vi "Unsubscribe from Topic.vi"(8 "error in (no error)":errorcluster, 9 "Topic":string, 10 "Subscriber Enq":refnum<class "Message Enqueuer.lvclass">, 11 "Publisher Actor in":refnum<class "Publisher Actor.lvclass">) -> (0 "error out":errorcluster, 3 "Publisher Actor out":refnum<class "Publisher Actor.lvclass">)   [LabVIEW 2021, in "Publisher Actor.lvclass"]
uses:
  Publisher Actor.lvclass
  <vilib>/ActorFramework/Message Enqueuer/Message Enqueuer.lvclass
  Publisher Actor.lvclass/Publisher Actor.ctl
  44acbf3b-423b-4e8c-ae4a-dc21de193688.vi
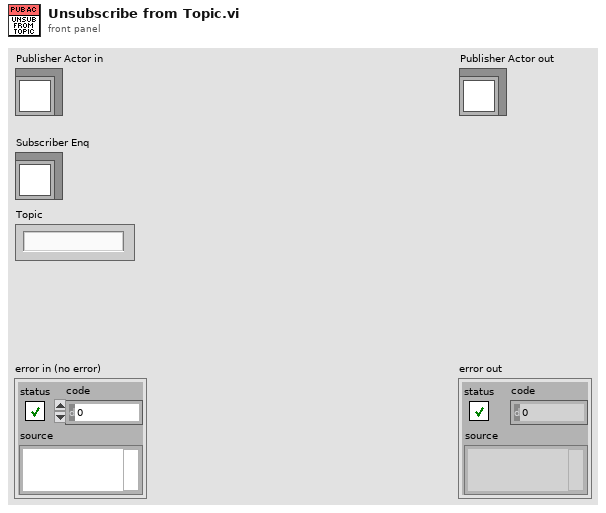
[diagram p1: front panel]
types:
  T1 = typedef "Context.ctl" = cluster{"Topic":string, "Source":string}
  T2 = map{T1, set{refnum<class "Message Enqueuer.lvclass">}}
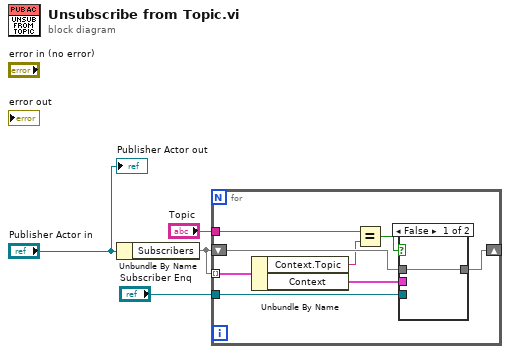
[diagram p0: block diagram]
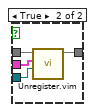
[diagram p2: hidden frame]
diagram:
  n1 = Unbundle By Name("Publisher Actor in") -> ("Subscribers"=w2:T2)
  n2 = for {
    tunnel: w2 -> [w9] mode=indexing
    tunnel: "Topic" -> [w5]
    shift-right: [w10] -> _
    shift-left: w2 -> [w11]
    tunnel: "Subscriber Enq" -> [w8]
    n3 = Unbundle By Name(w9) -> ("Context.Topic"=w6:string, "Context"=w7:T1)
    n4 = Equal?(x=w5, y=w6) -> (x = y?=w12:bool)
    n5 = case shown="False" w12 {
      tunnel: w11 -> [w13 w17]
      tunnel: [w13 w16] -> w10
      tunnel: w8 -> [_ w14]
      tunnel: w7 -> [_ w15]
      frame False {
      }
      frame True {
        n6 = call "Unregister.vim"("set element"=w14, "key"=w15, "map in"=w17) -> ("map out"=w16:T2)  [unwired: 6 in, 2 out]
      }
    }
  }
  "Publisher Actor out" <- "Publisher Actor in"
